vi "raw to tiff.vi"() -> ()   [LabVIEW 2012]
doc: "SciScan 1.2 160622"
uses:
  Custom Controls/file format type def tiff only.ctl
  Custom Controls/file format type def.ctl
  GFG/GFGnumericGet.vi
  GFG/GFGbooleanGet.vi
  save images/save channels to interleaved multi-tiff files.vi
  save images/save channels to separate multi-tiff files.vi
  save images/save channels to stacked multi-tiff files.vi
  save images/save channels to interleaved tiff series.vi
  save images/save channels to separate tiff series.vi
  save images/save channels to stacked tiff series.vi
  GFG/GFG library.lvlib
panel:
  out "Numeric Control":i32
  in  "file format":T1=enum."16bit multi-tiff (interleave)"
  in  "Path":path
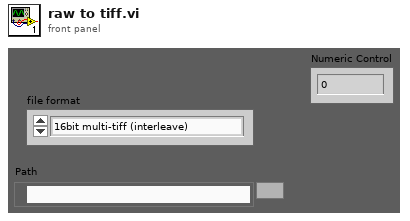
[diagram p1: front panel]
types:
  T1 = typedef "file format type def tiff only.ctl" = enum16{"16bit raw", "32bit raw", "16bit multi-tiff (interleave)", "16bit multi-tiff (separate)", "16bit multi-tiff (stacked)", "32bit multi-tiff (interleave)", "32bit multi-tiff (separate)", "32bit multi-tiff (stacked)", "16bit tiff series (interleave)", "16bit tiff series (separate)", "16bit tiff series (stacked)", "32bit tiff series (interleave)", "32bit tiff series (separate)", "32bit tiff series (stacked)"}
  T2 = typedef "file format type def.ctl" = enum16{"16bit raw", "32bit raw", "16bit multi-tiff (interleave)", "16bit multi-tiff (separate)", "16bit multi-tiff (stacked)", "32bit multi-tiff (interleave)", "32bit multi-tiff (separate)", "32bit multi-tiff (stacked)", "16bit tiff series (interleave)", "16bit tiff series (separate)", "16bit tiff series (stacked)", "32bit tiff series (interleave)", "32bit tiff series (separate)", "32bit tiff series (stacked)"}
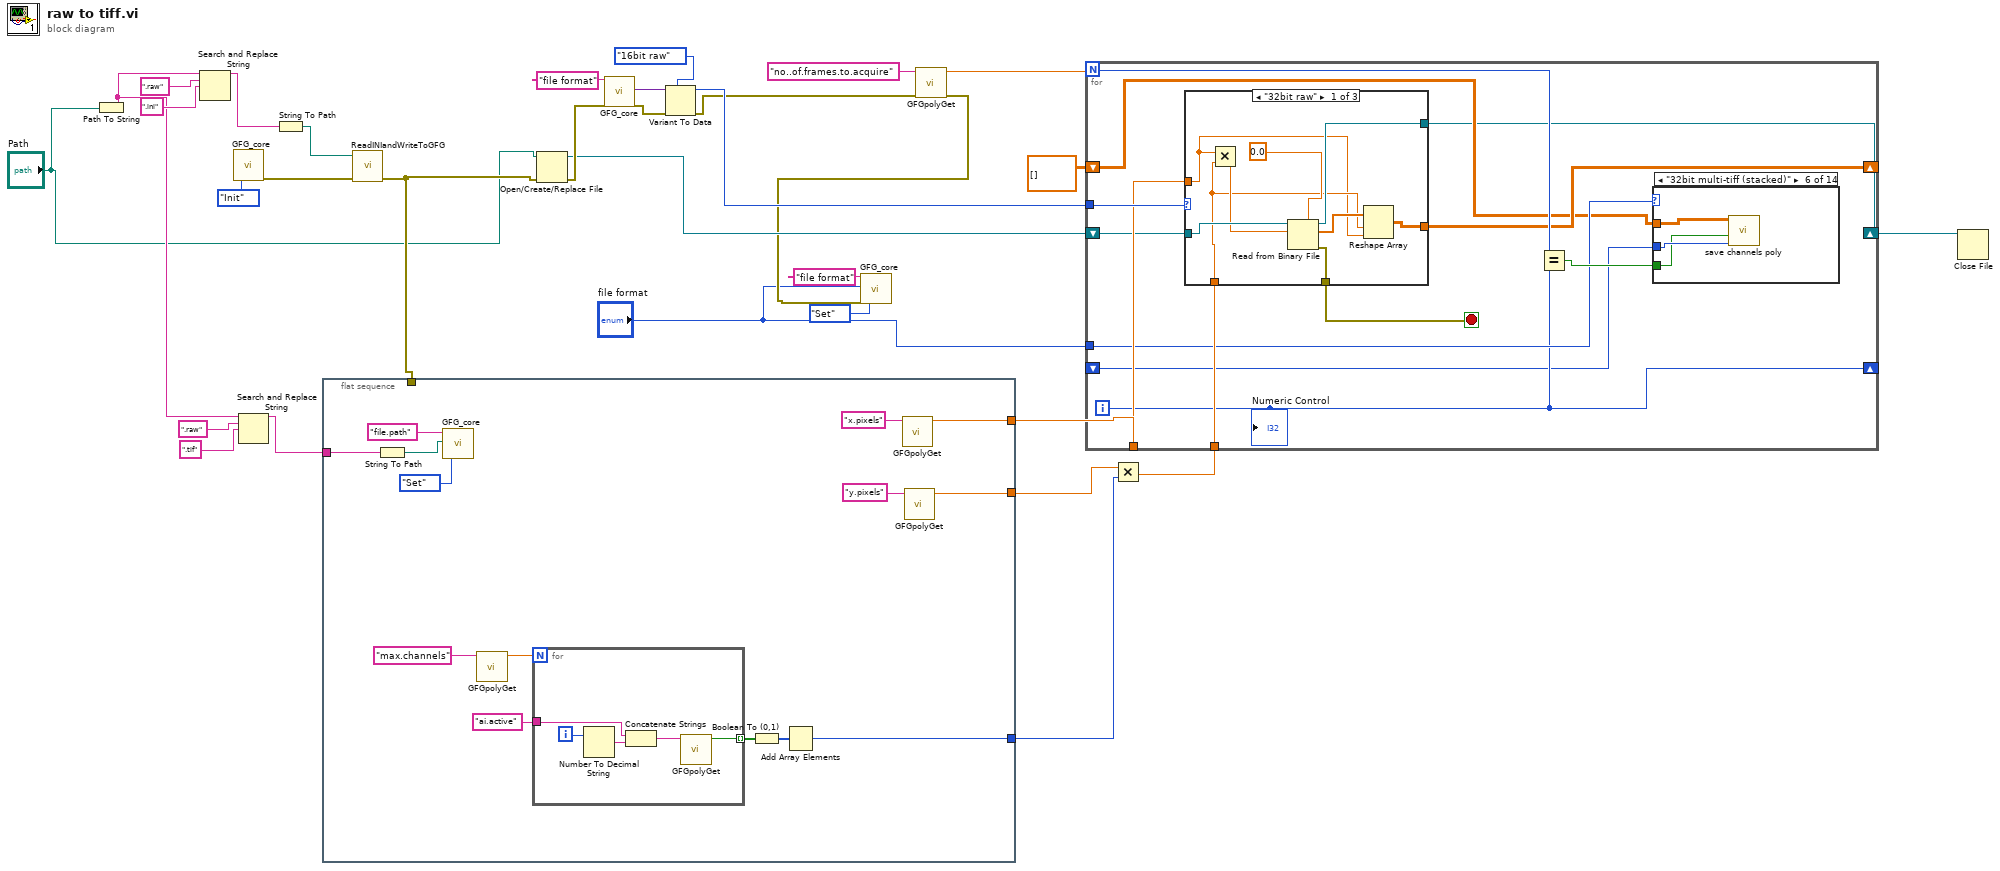
[diagram p0: block diagram]
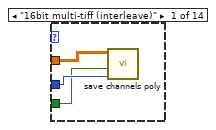
[diagram p2: hidden frame]
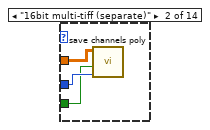
[diagram p3: hidden frame]
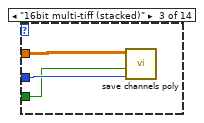
[diagram p4: hidden frame]
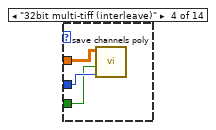
[diagram p5: hidden frame]
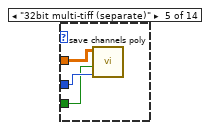
[diagram p6: hidden frame]
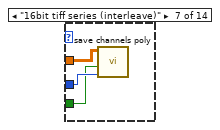
[diagram p7: hidden frame]
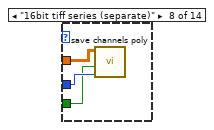
[diagram p8: hidden frame]
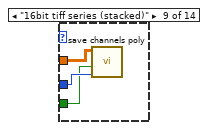
[diagram p9: hidden frame]
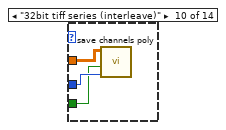
[diagram p10: hidden frame]
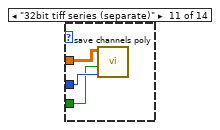
[diagram p11: hidden frame]
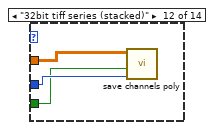
[diagram p12: hidden frame]
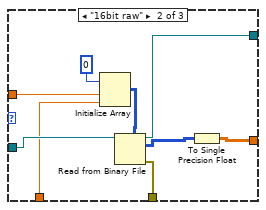
[diagram p15: hidden frame]
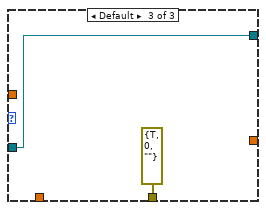
[diagram p16: hidden frame]
diagram:
  n1 = Path To String(path="Path") -> (string=w18:string)
  n2 = Search and Replace String(input string=w18, search string=".raw", replace string=".ini" ("replace string (\"\")")) -> (result string=w17:string)  [unwired: 5 in, 3 out]
  n3 = call "GFG_core.vi"("Action"=enum16{"Init", "Set", "Get"}."Init") -> ("error out"=w10:errorcluster)  [unwired: 12 in, 6 out]
  n4 = Search and Replace String(input string=w18, search string=".raw", replace string=".tif" ("replace string (\"\")")) -> (result string=w13:string)  [unwired: 5 in, 3 out]
  n5 = String To Path(string=w17) -> (path=w12:path)
  n6 = flat-sequence {
    tunnel: [w44] -> w27
    tunnel: [w38] -> w26
    tunnel: [w37] -> w24
    tunnel: w16 -> [_]
    tunnel: w13 -> [w35]
    frame #0 {
      n7 = String To Path(string=w35) -> (path=w33:path)
      n8 = call "GFG_core.vi"("Variable Name in"="file.path", "Variant in"=w33, "Action"=enum16{"Init", "Set", "Get"}."Set") -> ()  [unwired: 10 in, 7 out]
      n9 = call-poly "GFGpolyGet.vi"("Variable Name in"="max.channels") -> ("Numeric"=w42:dbl)  [unwired: 8 in, 2 out]
      n10 = for {
        N: w42 -> [_]
        tunnel: [w51] -> w40 mode=indexing
        tunnel: "ai.active" ("Variable Name in") -> [w50]
        i -> [w49]
        n11 = Number To Decimal String(number=w49) -> (decimal integer string=w48:string)  [unwired: 1 in]
        n12 = Concatenate Strings(w50, w48) -> (w47:string)
        n13 = call-poly "GFGpolyGet.vi"("Variable Name in"=w47) -> ("Boolean Value OUT"=w51:bool)  [unwired: 9 in, 1 out]
      }
      n14 = Boolean To (0,1)(Boolean=w40) -> (0, 1=w39:i16[])
      n15 = Add Array Elements(numeric array=w39) -> (sum=w38:i16)
      n16 = call-poly "GFGpolyGet.vi"("Variable Name in"="x.pixels") -> ("Numeric"=w37:dbl)  [unwired: 8 in, 2 out]
      n17 = call-poly "GFGpolyGet.vi"("Variable Name in"="y.pixels") -> ("Numeric"=w44:dbl)  [unwired: 8 in, 2 out]
    }
  }
  n18 = call "ReadINIandWriteToGFG.vi"("error in (no error)"=w10, "configuration file path"=w12) -> ("error out"=w16:errorcluster)  [unwired: 9 in]
  n19 = Open/Create/Replace File(file path (use dialog)="Path", error in=w16) -> (refnum out=w7:refnum<file>, error out=w29:errorcluster)  [unwired: 4 in, 1 out]
  n20 = call "GFG_core.vi"("Variable Name in"="file format", "error in (no error)"=w29) -> ("Variant Out"=w31:variant, "error out"=w15:errorcluster)  [unwired: 11 in, 5 out]
  n21 = Variant To Data(error in=w15, type=file_format_type_def."16bit raw" ("file format"), Variant=w31) -> (data=w28:T2, error out=w14:errorcluster)
  n22 = call-poly "GFGpolyGet.vi"("error in (no error)"=w14, "Variable Name in"="no..of.frames.to.acquire") -> ("error out"=w3:errorcluster, "Numeric"=w23:dbl)  [unwired: 7 in, 1 out]
  n23 = call "GFG_core.vi"("Variable Name in"="file format", "Variant in"="file format", "error in (no error)"=w3, "Action"=enum16{"Init", "Set", "Get"}."Set") -> ()  [unwired: 9 in, 7 out]
  n24 = Multiply(x=w27, y=w26) -> (x*y=w8:dbl)
  n25 = for {
    N: w23 -> [w60]
    tunnel: w28 -> [w64]
    tunnel: w8 -> [w63]
    tunnel: w24 -> [w62]
    tunnel: "file format" -> [w58]
    shift-right: [w57] -> _
    shift-left: _ -> [w56]
    shift-right: [w55] -> _
    shift-left: sgl[][] [] -> [w54]
    shift-right: [w53] -> w6
    shift-left: w7 -> [w52]
    i -> [w57]
    stop <- w61 stop-if-true
    n26 = case shown="\"32bit raw\"" w64 {
      tunnel: w52 -> [w109 w118 w119]
      tunnel: w63 -> [w103 w116 _]
      tunnel: w62 -> [w102 w115 _]
      tunnel: [w101 w112 _] -> w55
      tunnel: [w108 w111 errorcluster {"status"=TRUE, "code"=0, "source"=""} ("error out")] -> w61
      tunnel: [w107 w110 w119] -> w53
      frame "32bit raw" {
        n27 = Multiply(x=w102, y=w103) -> (x*y=w106:dbl)
        n28 = Read from Binary File(5:sgl 0.0, 10:w106, 11:w109) -> (0:w108:errorcluster, 2:w104:sgl[], 3:w107:refnum<file>)  [unwired: 3 in, 1 out]
        n29 = Reshape Array(w104, w103, w102) -> (w101:sgl[][])
      }
      frame "16bit raw" {
        n30 = Initialize Array(u16 0, w115, w116) -> (w114:u16[][])
        n31 = Read from Binary File(5:w114, 11:w118) -> (0:w111:errorcluster, 2:w113:u16[][], 3:w110:refnum<file>)  [unwired: 4 in, 1 out]
        n32 = To Single Precision Float(number=w113) -> (single precision float=w112:sgl[][])
      }
      frame Default {
      }
    }
    n33 = Equal?(x=w60, y=w57) -> (x = y?=w59:bool)
    n34 = case shown="\"32bit multi-tiff (stacked)\"" w58 {
      tunnel: w54 -> [w67 w70 w73 w76 w79 w82 w85 w88 w91 w94 w97 w100 _ _]
      tunnel: w56 -> [w66 w69 w72 w75 w78 w81 w84 w87 w90 w93 w96 w99 _ _]
      tunnel: w59 -> [w65 w68 w71 w74 w77 w80 w83 w86 w89 w92 w95 w98 _ _]
      frame "16bit multi-tiff (interleave)" {
        n35 = call-poly "save channels poly.vi"("frame number in"=w66, "last frame"=w65, "image data in"=w67) -> ()  [unwired: 9 in]
      }
      frame "16bit multi-tiff (separate)" {
        n36 = call-poly "save channels poly.vi"("frame number in"=w69, "last frame"=w68, "image data in"=w70) -> ()  [unwired: 9 in]
      }
      frame "16bit multi-tiff (stacked)" {
        n37 = call-poly "save channels poly.vi"("frame number in"=w72, "last frame"=w71, "image data in"=w73) -> ()  [unwired: 9 in]
      }
      frame "32bit multi-tiff (interleave)" {
        n38 = call-poly "save channels poly.vi"("frame number in"=w75, "last frame"=w74, "image data in"=w76) -> ()  [unwired: 9 in]
      }
      frame "32bit multi-tiff (separate)" {
        n39 = call-poly "save channels poly.vi"("frame number in"=w78, "last frame"=w77, "image data in"=w79) -> ()  [unwired: 9 in]
      }
      frame "32bit multi-tiff (stacked)" {
        n40 = call-poly "save channels poly.vi"("frame number in"=w81, "last frame"=w80, "image data in"=w82) -> ()  [unwired: 9 in]
      }
      frame "16bit tiff series (interleave)" {
        n41 = call-poly "save channels poly.vi"("frame number in"=w84, "last frame"=w83, "image data in"=w85) -> ()  [unwired: 9 in]
      }
      frame "16bit tiff series (separate)" {
        n42 = call-poly "save channels poly.vi"("frame number in"=w87, "last frame"=w86, "image data in"=w88) -> ()  [unwired: 9 in]
      }
      frame "16bit tiff series (stacked)" {
        n43 = call-poly "save channels poly.vi"("frame number in"=w90, "last frame"=w89, "image data in"=w91) -> ()  [unwired: 9 in]
      }
      frame "32bit tiff series (interleave)" {
        n44 = call-poly "save channels poly.vi"("frame number in"=w93, "last frame"=w92, "image data in"=w94) -> ()  [unwired: 9 in]
      }
      frame "32bit tiff series (separate)" {
        n45 = call-poly "save channels poly.vi"("frame number in"=w96, "last frame"=w95, "image data in"=w97) -> ()  [unwired: 9 in]
      }
      frame "32bit tiff series (stacked)" {
        n46 = call-poly "save channels poly.vi"("frame number in"=w99, "last frame"=w98, "image data in"=w100) -> ()  [unwired: 9 in]
      }
      frame "32bit raw" {
      }
      frame "16bit raw" {
      }
    }
    "Numeric Control" <- w57
  }
  n47 = Close File(refnum=w6) -> ()  [unwired: 1 in, 2 out]
